vi "Write UI Ref.vi"(8 "error in (no error)":errorcluster, 10 "UI Ref":refnum<vi>, 11 "Actor wUI in":refnum<class "Actor wUI.lvclass">) -> (0 "error out":errorcluster, 3 "Actor wUI out":refnum<class "Actor wUI.lvclass">)   [LabVIEW 2017, in "Framework.lvlib" / "Actor wUI.lvclass"]
uses:
  Actor wUI.lvclass
  Actor wUI.lvclass/Actor wUI.ctl
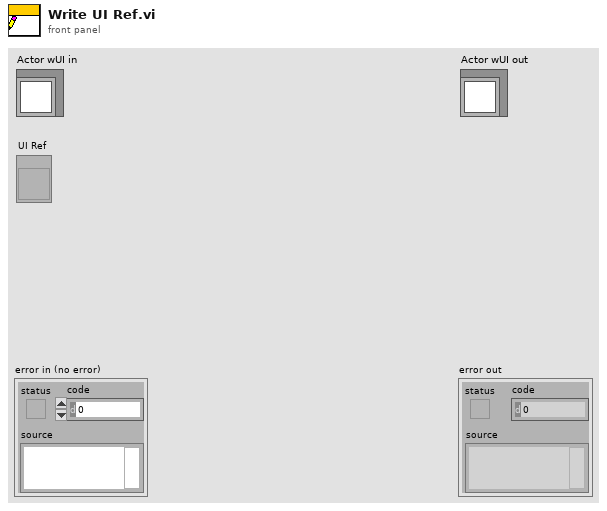
[diagram p1: front panel]
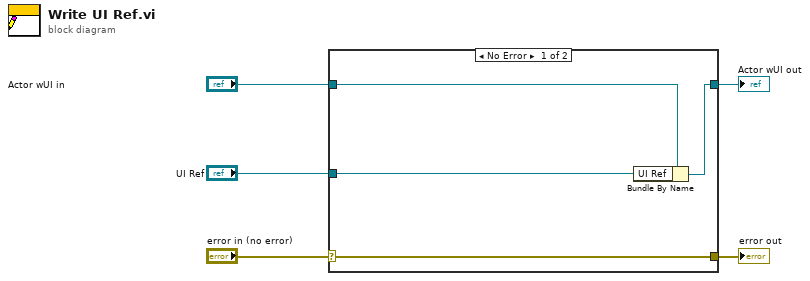
[diagram p0: block diagram]
diagram:
  n1 = case shown="No Error" "error in (no error)" {
    selector: "error in (no error)" -> [w9 w10]
    tunnel: [w9 w10] -> w4
    tunnel: [w7 w11] -> w2
    tunnel: "Actor wUI in" -> [w8 w11]
    tunnel: "UI Ref" -> [w6 _]
    frame No Error {
      n2 = Bundle By Name(cluster=w8, "UI Ref"=w6) -> (w7:refnum<class "Actor wUI.lvclass">)
    }
    frame Error {
    }
  }
  "error out" <- w4
  "Actor wUI out" <- w2
